vi "Unknown Error Code constant.vi"() -> (3 "AWS Unknown Error Code value":i32)   [LabVIEW 2015, in "NI_AWS_Core.lvlib" / "HTTP Request.lvclass"]
uses:
  HTTP Request.lvclass
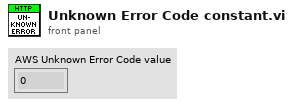
[diagram p1: front panel]
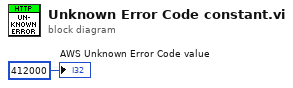
[diagram p0: block diagram]
diagram:
  "AWS Unknown Error Code value" <- 412000
